vi "Generate ConfigFile Path.vi"() -> (0 "ConfigFile path":path)   [LabVIEW 2018, in "FPGA Addon DMA Channels Basic System Tests.lvclass"]
uses:
  FPGA Addon DMA Channels Basic System Tests.lvclass
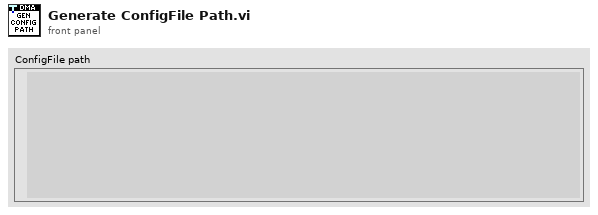
[diagram p1: front panel]
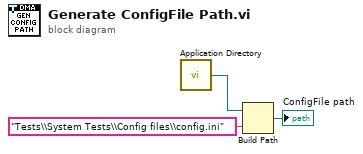
[diagram p0: block diagram]
diagram:
  n1 = call <vilib>:"Application Directory.vi"() -> ("Application Directory"=w3:path)
  n2 = Build Path(base path=w3, name or relative path="Tests\\System Tests\\Config files\\config.ini") -> (appended path=→"ConfigFile path":path)
